vi "Reignite.vi"(8 "error in (no error)":errorcluster, 10 "Relight State":string, 11 "BaseProducer in":refnum<class "BaseProducer.lvclass">) -> (0 "error out":errorcluster, 3 "BaseProducer out":refnum<class "BaseProducer.lvclass">)   [LabVIEW 2013, in "BaseProducer.lvclass"]
doc: "This method returns the combustor to the re-ignition state."
uses:
  BaseProducer.lvclass
  BaseProducer.lvclass/BaseProducer.ctl
  <vilib>/DAQmx/write.llb/DAQmx Write (Analog 1D DBL NChan 1Samp).vi
  <vilib>/DAQmx/miscellaneous.llb/DAQmx Fill In Error Info.vi
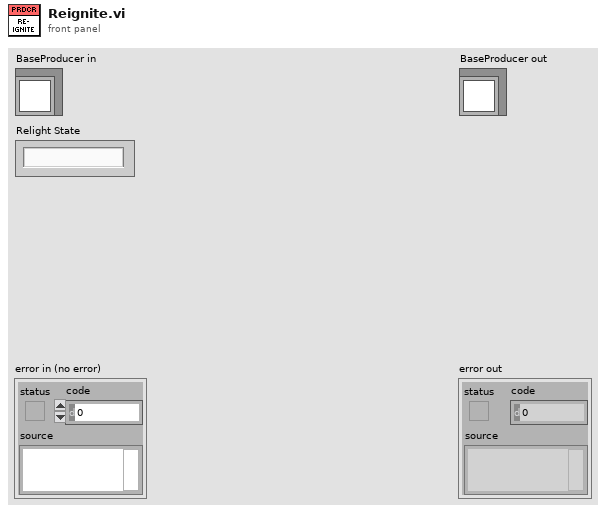
[diagram p1: front panel]
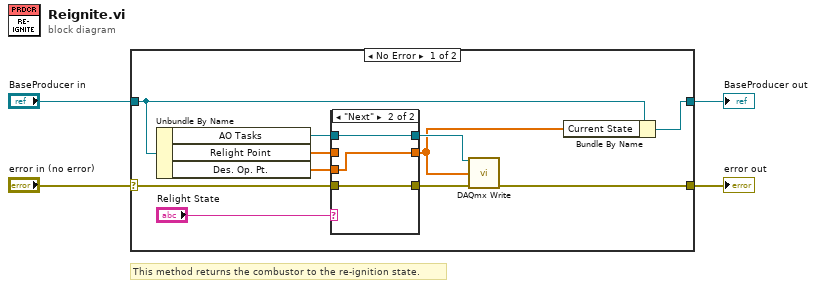
[diagram p0: block diagram]
diagram:
  # "This method returns the combustor to the re-ignition state."
  n1 = case shown="No Error" "error in (no error)" {
    selector: "error in (no error)" -> [w8 w23]
    tunnel: [w15 w23] -> w3
    tunnel: [w13 w22] -> w1
    tunnel: "BaseProducer in" -> [w14 w22]
    frame No Error {
      n2 = Unbundle By Name(w14) -> ("AO Tasks"=w11:refnum<k21>, "Relight Point"=w10:dbl[], "Des. Op. Pt."=w9:dbl[])
      n3 = case shown="\"Next\"" "Relight State" {
        tunnel: w11 -> [w16 w21]
        tunnel: w10 -> [w17 _]
        tunnel: w9 -> [_ w20]
        tunnel: w8 -> [w18 w19]
        tunnel: [w18 w19] -> w7
        tunnel: [w17 w20] -> w5
        tunnel: [w16 w21] -> w6
        frame "Skip", Default {
        }
        frame "Next" {
        }
      }
      n4 = call-poly <vilib>:"DAQmx Write.vi"("task/channels in"=w6, "data"=w5, "error in"=w7) -> ("error out"=w15:errorcluster)  [unwired: 10 in, 2 out]
      n5 = Bundle By Name(cluster=w14, "Current State"=w5) -> (w13:refnum<class "BaseProducer.lvclass">)
    }
    frame Error {
    }
  }
  "error out" <- w3
  "BaseProducer out" <- w1
